vi "Kinect Get Depth Image.vi"(8 "error in (no error)":errorcluster) -> (0 "error out":errorcluster, 3 "Depth Image":T1)   [LabVIEW 2011]
uses:
  <vilib>/vision/Image Controls.llb/IMAQ Image.ctl
  Kinect Global Status.vi
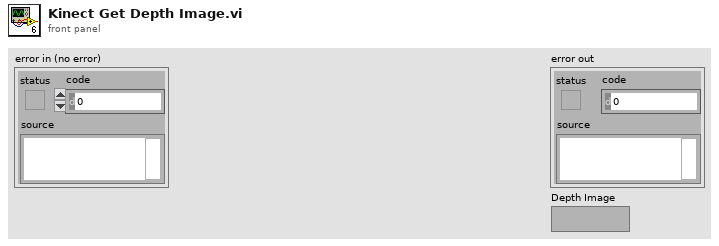
[diagram p1: front panel]
types:
  T1 = typedef "IMAQ Image.ctl" = refnum<image>
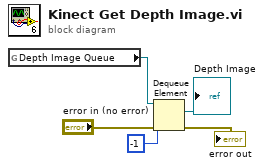
[diagram p0: block diagram]
diagram:
  n1 = global read "Kinect Global Status.vi" "Depth Image Queue"() -> (w5:refnum<queue>)
  n2 = Dequeue Element(queue=w5, timeout in ms (-1)=-1, error in (no error)="error in (no error)") -> (element=→"Depth Image":T1, error out=→"error out":errorcluster)  [unwired: 2 out]
